vi "Transparency.vi"() -> ()   [LabVIEW 2018]
uses:
  <vilib>/Analysis/3filter.llb/Filter Passband Type.ctl
  <vilib>/DAQmx/write.llb/DAQmx Write (Analog 1D DBL NChan 1Samp).vi
  <vilib>/DAQmx/read.llb/DAQmx Read (Analog 1D DBL NChan 1Samp).vi
  <vilib>/DAQmx/create/channels.llb/DAQmx Create Channel (AO-Voltage-Basic).vi
  <vilib>/DAQmx/create/channels.llb/DAQmx Create Channel (AI-Voltage-Basic).vi
  <vilib>/DAQmx/miscellaneous.llb/DAQmx Fill In Error Info.vi
  <vilib>/ptbypt/NI_PtbyPt.lvlib
  <vilib>/Analysis/NI_AALBase.lvlib
panel:
  out "Measured Acceleration":dbl(graph)
  in  "K":dbl
  in  "Force filter Y/N":bool
  out "Desired Vel":dbl(graph)
  out "Desired acc":dbl(graph)
  in  "I_app_wall":dbl
  in  "I_app_transp":dbl=1e-06 min=1e-06 max=0.1 step=1e-06
  in  "B":dbl
  out "Velocity Meas":dbl(graph)
  in  "Vel Fil Y/N":bool
  in  "Loop Frequency":dbl
  out "Position Measured":dbl(graph)
  in  "Pos Fil Y/N":bool
  out "Force measure":dbl(graph)
  in  "stop":bool
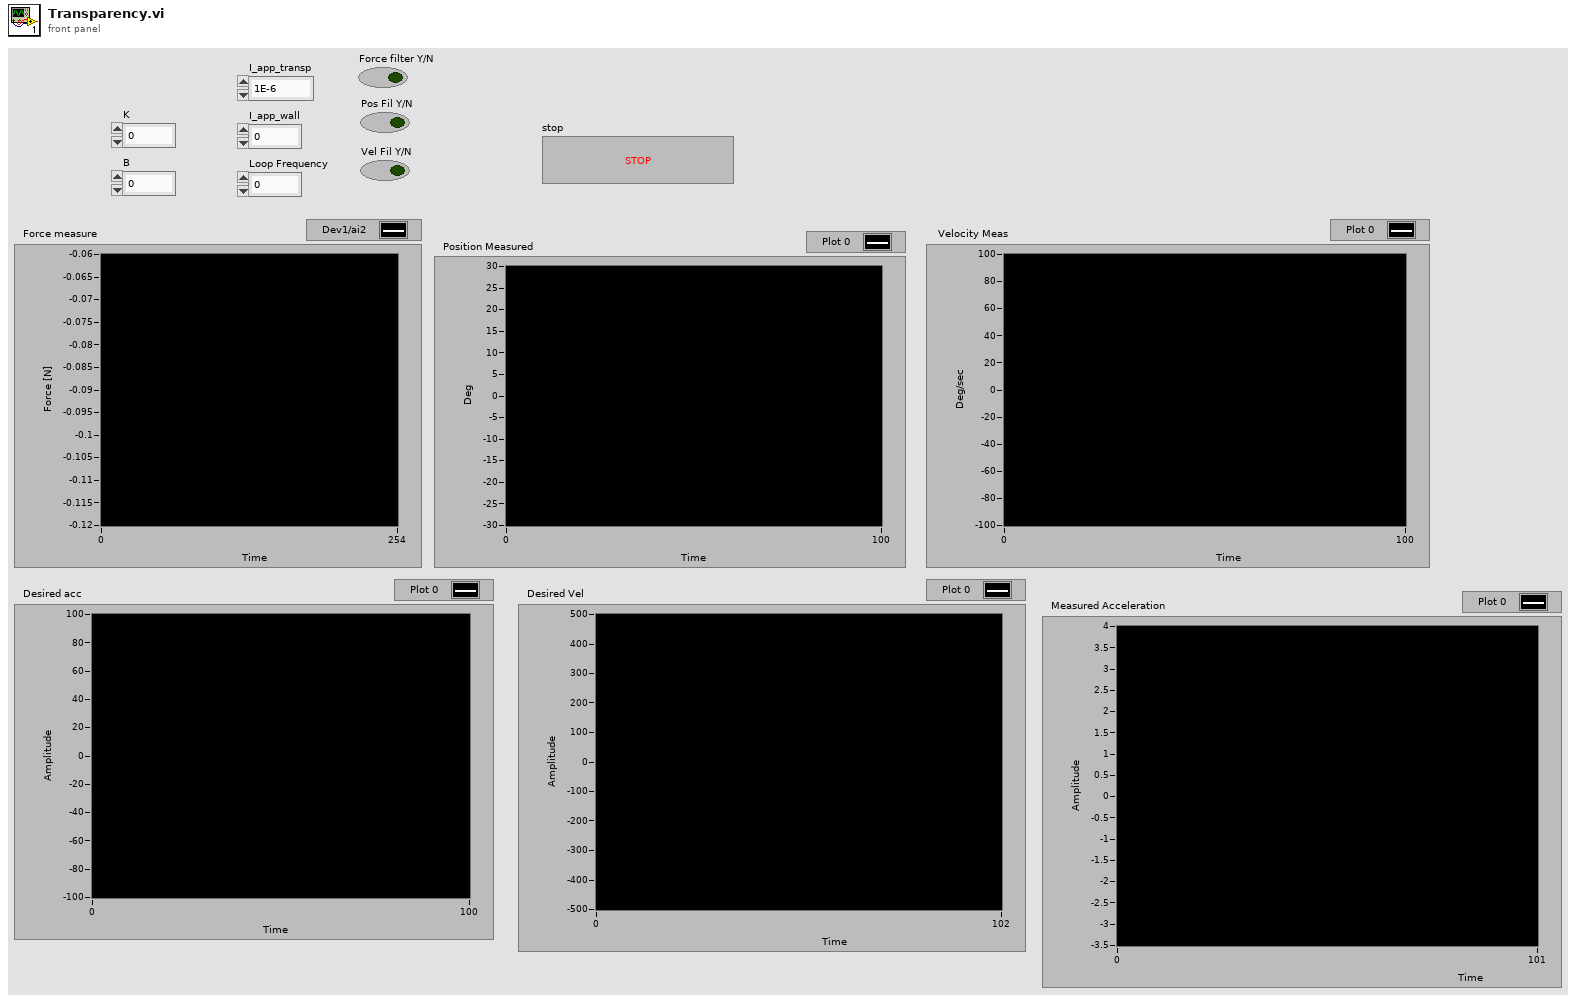
[diagram p1: front panel]
types:
  T1 = typedef "NI_AALBase.lvlib/Filter Passband Type.ctl" = enum32{"Lowpass", "Highpass", "Bandpass", "Bandstop"}
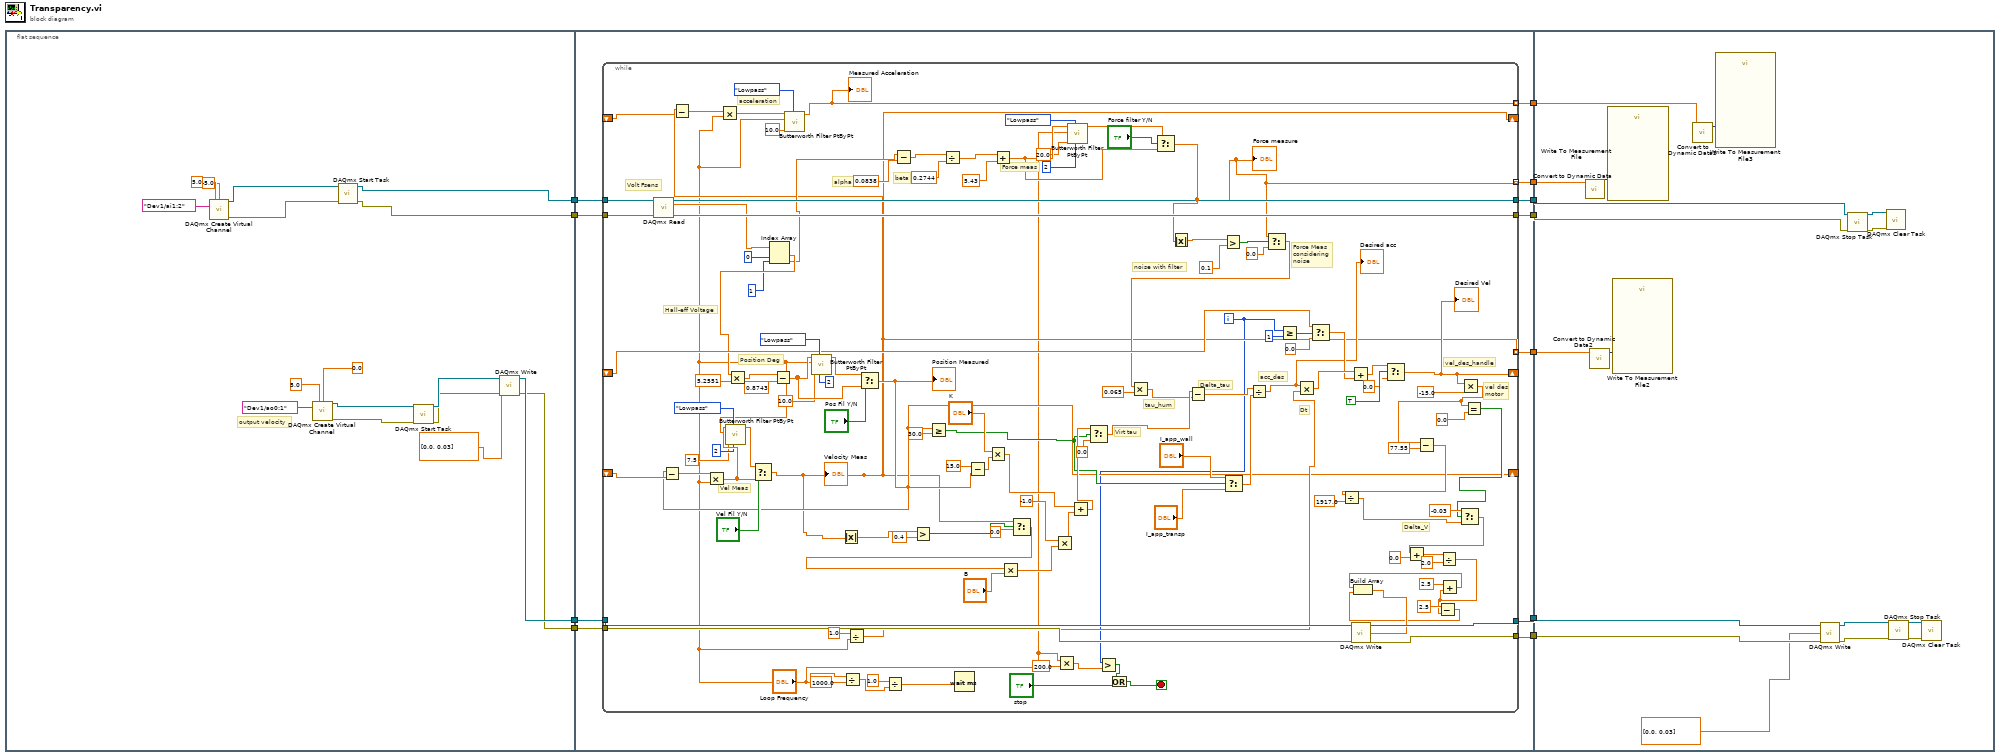
[diagram p0: block diagram]
diagram:
  n1 = flat-sequence {
    tunnel: [w25] -> w9
    tunnel: [w22] -> w7
    tunnel: [w12] -> w5
    tunnel: [w13] -> w4
    tunnel: [w39] -> w11
    tunnel: [w38] -> w10
    tunnel: w9 -> [w37]
    tunnel: [w36] -> w8
    tunnel: w7 -> [w35]
    tunnel: [w34] -> w6
    tunnel: w5 -> [w33]
    tunnel: w4 -> [w32]
    tunnel: [w31] -> w3
    tunnel: [w30] -> w2
    tunnel: [w29] -> w1
    tunnel: w11 -> [w178]
    tunnel: w10 -> [w176]
    tunnel: w8 -> [w172]
    tunnel: w6 -> [w170]
    tunnel: w3 -> [w167]
    tunnel: w2 -> [w165]
    tunnel: w1 -> [w163]
    frame #0 {
      # "output velocity"
      n2 = call-poly <vilib>:"DAQmx Create Virtual Channel.vi"("maximum value"=5.0, "minimum value"=-5.0, "physical channels"=tag "Dev1/ai1:2") -> ("task out"=w19:refnum<k21>, "error out"=w18:errorcluster)  [unwired: 11 in]
      n3 = call-poly <vilib>:"DAQmx Create Virtual Channel.vi"("maximum value"=5.0, "minimum value"=0.0, "physical channels"=tag "Dev1/ao0:1") -> ("task out"=w27:refnum<k21>, "error out"=w24:errorcluster)  [unwired: 11 in]
      n4 = call <vilib>:"DAQmx Start Task.vi"("task/channels in"=w19, "error in"=w18) -> ("task out"=w13:refnum<k21>, "error out"=w12:errorcluster)  [unwired: 12 in]
      n5 = call <vilib>:"DAQmx Start Task.vi"("task/channels in"=w27, "error in"=w24) -> ("task out"=w26:refnum<k21>, "error out"=w23:errorcluster)  [unwired: 12 in]
      n6 = call-poly <vilib>:"DAQmx Write.vi"("task/channels in"=w26, "data"=dbl[] [0.0, 0.03], "error in"=w23) -> ("task out"=w25:refnum<k21>, "error out"=w22:errorcluster)  [unwired: 10 in, 1 out]
    }
    frame #1 {
      n7 = while {
        tunnel: [w161] -> w39
        tunnel: [w160] -> w38
        tunnel: w37 -> [w156]
        tunnel: [w155] -> w36
        tunnel: w35 -> [w154]
        tunnel: [w153] -> w34
        shift-right: [w59] -> _
        shift-left: _ -> [w86]
        tunnel: w33 -> [w129]
        tunnel: w32 -> [w128]
        shift-right: [w66] -> _
        shift-left: _ -> [w112]
        tunnel: [w55] -> w31 mode=indexing
        tunnel: [w54] -> w30 mode=indexing
        shift-right: [w54] -> _
        shift-left: _ -> [w53]
        tunnel: [w41] -> w29 mode=indexing
        i -> [w48]
        stop <- w42 stop-if-true
        # "acceleration"
        # "vel des\nmotor"
        # "Dt"
        # "Force Meas\nconsidering\nnoise"
        # "noise with filter"
        # "Force meas"
        # "Virt tau"
        # "Vel Meas"
        # "Hall-eff Voltage"
        # "Delta_tau"
        # "tau_hum"
        # "vel_des_handle"
        # "Delta_V"
        # "acc_des"
        # "Position Deg"
        # "Volt Fsens"
        # "beta"
        # "alpha"
        n8 = call-poly <vilib>:"DAQmx Read.vi"("task/channels in"=w128, "error in"=w129) -> ("task out"=w161:refnum<k21>, "data"=w130:dbl[], "error out"=w160:errorcluster)  [unwired: 11 in]
        n9 = Index Array(array=w130, index #1=0 ("index"), index #2=1 ("index")) -> (element #1=w94:dbl, element #2=w93:dbl)
        n10 = Multiply(x=w94, y=5.2551) -> (x*y=w151:dbl)
        n11 = Subtract(x=w151, y=0.8743) -> (x-y=w147:dbl)
        n12 = call <vilib>:"Butterworth Filter PtByPt.vi"("order"=2, "filter type"=Filter_Passband_Type."Lowpass", "low cutoff freq: fl"=10.0, "sampling freq: fs"="Loop Frequency", "x"=w147) -> ("Filtered x"=w148:dbl)  [unwired: 4 in, 1 out]
        n13 = Divide(x="Loop Frequency", y=1000.0) -> (x/y=w142:dbl)
        n14 = Divide(x=1.0, y="Loop Frequency") -> (x/y=w116:dbl)
        n15 = Select(t=w148, s="Pos Fil Y/N", f=w147) -> (s? t:f=w59:dbl)
        "Position Measured" <- w59
        n16 = Subtract(x=w59, y=w86) -> (x-y=w139:dbl)
        n17 = Multiply(x=w139, y="Loop Frequency") -> (x*y=w137:dbl)
        n18 = call <vilib>:"Butterworth Filter PtByPt.vi"("order"=2, "filter type"=Filter_Passband_Type."Lowpass", "low cutoff freq: fl"=7.5, "sampling freq: fs"="Loop Frequency", "x"=w137) -> ("Filtered x"=w136:dbl)  [unwired: 4 in, 1 out]
        n19 = Select(t=w136, s="Vel Fil Y/N", f=w137) -> (s? t:f=w54:dbl)
        "Velocity Meas" <- w54
        n20 = Subtract(x=w54, y=w53) -> (x-y=w52:dbl)
        n21 = Multiply(x=w52, y="Loop Frequency") -> (x*y=w51:dbl)
        n22 = call <vilib>:"Butterworth Filter PtByPt.vi"("filter type"=Filter_Passband_Type."Lowpass", "low cutoff freq: fl"=10.0, "sampling freq: fs"="Loop Frequency", "x"=w51) -> ("Filtered x"=w41:dbl)  [unwired: 5 in, 1 out]
        "Measured Acceleration" <- w41
        n23 = Absolute Value(x=w54) -> (abs(x)=w85:dbl)
        n24 = Divide(x=1.0, y=w142) -> (x/y=w127:dbl)
        n25 = Subtract(x=w93, y=0.0838) -> (x-y=w159:dbl)
        n26 = Greater?(x=w85, y=0.4) -> (0:w83:bool)
        n27 = Greater Or Equal?(x=w59, y=30.0) -> (x >= y?=w61:bool)
        n28 = Divide(x=w159, y=0.2744) -> (x/y=w107:dbl)
        n29 = Wait (ms)(milliseconds to wait=w127) -> ()  [unwired: 1 out]
        n30 = Subtract(x=15.0, y=w59) -> (x-y=w75:dbl)
        n31 = Multiply(x="K", y=w75) -> (x*y=w73:dbl)
        n32 = Add(x=w107, y=5.43) -> (x+y=w103:dbl)
        n33 = Select(t=w54, s=w83, f=0.0) -> (s? t:f=w81:dbl)
        n34 = Multiply(x=w81, y="B") -> (x*y=w89:dbl)
        n35 = Multiply(x=-1.0, y=w89) -> (x*y=w77:dbl)
        n36 = Multiply(x="Loop Frequency", y=200.0) -> (x*y=w45:dbl)
        n37 = call <vilib>:"Butterworth Filter PtByPt.vi"("order"=2, "filter type"=Filter_Passband_Type."Lowpass", "low cutoff freq: fl"=20.0, "sampling freq: fs"="Loop Frequency", "x"=w103) -> ("Filtered x"=w104:dbl)  [unwired: 4 in, 1 out]
        n38 = Add(x=w73, y=w77) -> (x+y=w72:dbl)
        n39 = Select(t=w72, s=w61, f=0.0) -> (s? t:f=w109:dbl)
        n40 = Greater?(x=w48, y=w45) -> (0:w44:bool)
        n41 = Or(x=w44, y="stop") -> (x .or. y?=w42:bool)
        n42 = Select(t=w104, s="Force filter Y/N", f=w103) -> (s? t:f=w55:dbl)
        "Force measure" <- w55
        n43 = Absolute Value(x=w55) -> (abs(x)=w95:dbl)
        n44 = Greater?(x=w95, y=0.1) -> (0:w63:bool)
        n45 = Select(t="I_app_wall", s=w61, f="I_app_transp") -> (s? t:f=w117:dbl)
        n46 = Select(t=w55, s=w63, f=0.0) -> (s? t:f=w96:dbl)
        n47 = Multiply(x=w96, y=0.065) -> (x*y=w106:dbl)
        n48 = Subtract(x=w109, y=w106) -> (x-y=w90:dbl)
        n49 = Divide(x=w90, y=w117) -> (x/y=w105:dbl)
        "Desired acc" <- w105
        n50 = Greater Or Equal?(x=w48, y=1) -> (x >= y?=w114:bool)
        n51 = Multiply(x=w105, y=w116) -> (x*y=w115:dbl)
        n52 = Select(t=w112, s=w114, f=0.0) -> (s? t:f=w110:dbl)
        n53 = Add(x=w115, y=w110) -> (x+y=w57:dbl)
        n54 = Select(t=w57, s=TRUE, f=0.0) -> (s? t:f=w66:dbl)
        "Desired Vel" <- w66
        n55 = Multiply(x=w66, y=-15.0) -> (x*y=w62:dbl)
        n56 = Subtract(x=w62, y=77.55) -> (x-y=w79:dbl)
        n57 = Divide(x=w79, y=1917.0) -> (x/y=w40:dbl)
        n58 = Equal?(x=w62, y=0.0) -> (x = y?=w60:bool)
        n59 = Select(t=-0.03, s=w60, f=w40) -> (s? t:f=w67:dbl)
        n60 = Add(x=w67, y=0.0) -> (x+y=w124:dbl)
        n61 = Divide(x=w124, y=2.0) -> (x/y=w120:dbl)
        n62 = Subtract(x=2.5, y=w120) -> (x-y=w69:dbl)
        n63 = Add(x=2.5, y=w120) -> (x+y=w70:dbl)
        n64 = Build Array(w70, w69) -> (w82:dbl[])
        n65 = call-poly <vilib>:"DAQmx Write.vi"("task/channels in"=w156, "data"=w82, "error in"=w154) -> ("task out"=w155:refnum<k21>, "error out"=w153:errorcluster)  [unwired: 10 in, 1 out]
      }
    }
    frame #2 {
      n66 = call "Convert to Dynamic Data"("Array"=w167) -> ("Dynamic Data Type"=w166:dynamicdata)  [unwired: 3 in]
      n67 = call "Convert to Dynamic Data2"("Array"=w165) -> ("Dynamic Data Type"=w164:dynamicdata)  [unwired: 3 in]
      n68 = call "Write To Measurement File"("Signals"=w166) -> ()  [unwired: 16 in, 3 out]
      n69 = call "Write To Measurement File2"("Signals"=w164) -> ()  [unwired: 16 in, 3 out]
      n70 = call "Convert to Dynamic Data3"("Array"=w163) -> ("Dynamic Data Type"=w162:dynamicdata)  [unwired: 3 in]
      n71 = call "Write To Measurement File3"("Signals"=w162) -> ()  [unwired: 16 in, 3 out]
      n72 = call-poly <vilib>:"DAQmx Write.vi"("task/channels in"=w172, "data"=dbl[] [0.0, 0.03], "error in"=w170) -> ("task out"=w171:refnum<k21>, "error out"=w169:errorcluster)  [unwired: 10 in, 1 out]
      n73 = call <vilib>:"DAQmx Stop Task.vi"("task/channels in"=w178, "error in"=w176) -> ("task out"=w177:refnum<k21>, "error out"=w175:errorcluster)  [unwired: 12 in]
      n74 = call <vilib>:"DAQmx Clear Task.vi"("task in"=w177, "error in"=w175) -> ()  [unwired: 13 in, 1 out]
      n75 = call <vilib>:"DAQmx Stop Task.vi"("task/channels in"=w171, "error in"=w169) -> ("task out"=w174:refnum<k21>, "error out"=w173:errorcluster)  [unwired: 12 in]
      n76 = call <vilib>:"DAQmx Clear Task.vi"("task in"=w174, "error in"=w173) -> ()  [unwired: 13 in, 1 out]
    }
  }
